vi "subsystem_getEvent_SummaryState.vi"(8 "error in (no error)":errorcluster, 11 "ProgrammaticInitialization in":refnum<class "ProgrammaticInitialization.lvclass">) -> (0 "error out":errorcluster, 2 "logevent_SummaryState":T1, 3 "ProgrammaticInitialization out":refnum<class "ProgrammaticInitialization.lvclass">)   [LabVIEW 2016, in "ProgrammaticInitialization.lvclass"]
uses:
  ProgrammaticInitialization.lvclass
  ts_sallv_FiberSpectrograph/DataTypes/logevent_summaryState.ctl
  ts_sallv_FiberSpectrograph/DataTypes/logevent_errorCode.ctl
  ts_sallv_FiberSpectrograph/SALLV_FiberSpectrograph.lvlib
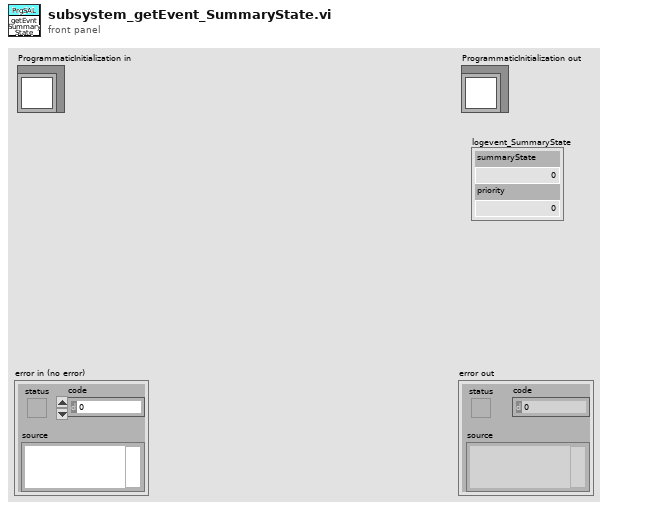
[diagram p1: front panel]
types:
  T1 = typedef "SALLV_FiberSpectrograph.lvlib/logevent_summaryState.ctl" = cluster{"summaryState":i32, "priority":i32}
  T2 = typedef "SALLV_FiberSpectrograph.lvlib/logevent_errorCode.ctl" = cluster{"errorCode":i32, "priority":i32}
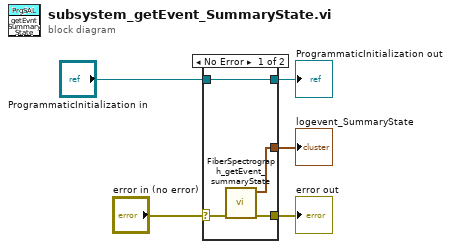
[diagram p0: block diagram]
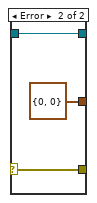
[diagram p2: hidden frame]
diagram:
  n1 = case shown="No Error" "error in (no error)" {
    selector: "error in (no error)" -> [w6 w12]
    tunnel: [w7 w12] -> w4
    tunnel: [w9 w11] -> w2
    tunnel: "ProgrammaticInitialization in" -> [w9 w11]
    tunnel: [w8 T2 {"errorCode"=0, "priority"=0} ("logevent_ErrorCode_Ctl out")] -> w1
    frame No Error {
      n2 = call "FiberSpectrograph_getEvent_summaryState.vi"("error in (no error)"=w6) -> ("error out"=w7:errorcluster, "logevent_summaryState_Ctl out"=w8:T1)  [unwired: 8 in, 1 out]
    }
    frame Error {
    }
  }
  "error out" <- w4
  "ProgrammaticInitialization out" <- w2
  "logevent_SummaryState" <- w1
